vi "Build Metric Values.vi"(7 "TimingEngine":T1, 8 "error in (no error)":errorcluster, 10 "Waveform Array":sgl[][](array[numeric]), 11 "DAQ Task":refnum<class "DAQ Task.lvclass">) -> (0 "error out":errorcluster, 1 "Modbus Values":dbl[](array[numeric]), 2 "Ch Metrics":dbl[](array[numeric]), 3 "DAQ Task":refnum<class "DAQ Task.lvclass">)   [LabVIEW 2012, in "Data Acquisition.lvlib" / "DAQ Task.lvclass"]
uses:
  DAQ Task.lvclass
  Common/Controls/TE_Designator.ctl
  DAQ Task.lvclass/DAQ Task.ctl
  Measurements/Class Channel/Channel.lvclass
  Measurements/Class Channel/Read ToModBus.vi
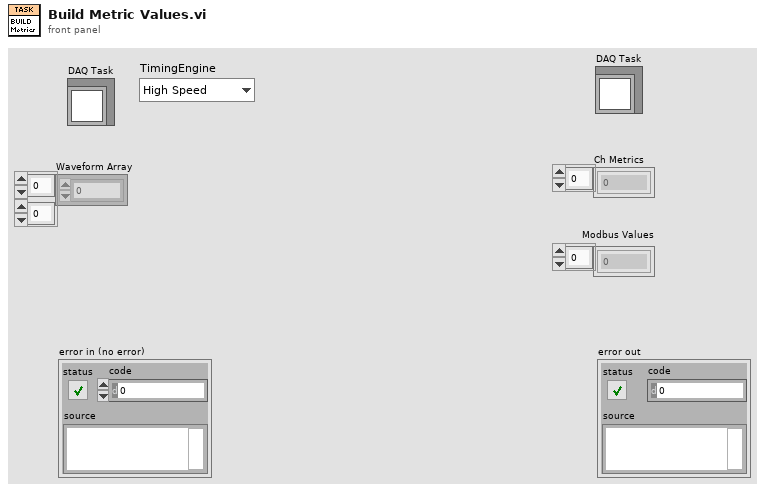
[diagram p1: front panel]
types:
  T1 = typedef "TE_Designator.ctl" = enum16{"High Speed", "Low Speed"}
  T2 = typedef "Group Timing Info.ctl" = cluster{"Rate":dbl, "ReadBlk":i32}
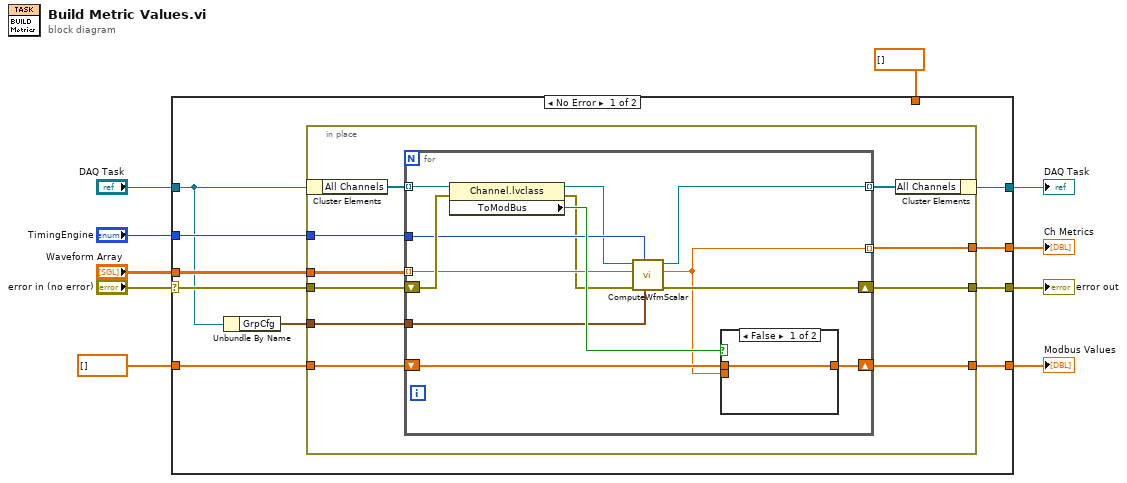
[diagram p0: block diagram]
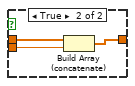
[diagram p2: hidden frame]
diagram:
  n1 = case shown="No Error" "error in (no error)" {
    selector: "error in (no error)" -> [w18 w50]
    tunnel: [w16 w48] -> w10
    tunnel: "Waveform Array" -> [w20 _]
    tunnel: "DAQ Task" -> [w12 w49]
    tunnel: [w15 w49] -> w7
    tunnel: [w19 w50] -> w6
    tunnel: "TimingEngine" -> [w17 _]
    tunnel: dbl[] [] -> [_ w48]
    tunnel: dbl[] [] -> [w14 _]
    tunnel: [w13 w48] -> w1
    frame No Error {
      n2 = Unbundle By Name(w12) -> ("GrpCfg"=w11:T2)
      n3 = in-place {
        in-place-border: w20 -> [w30]
        in-place-border: [w29] -> w19
        in-place-border: w18 -> [w28]
        in-place-border: w17 -> [w27]
        in-place-border: [w26] -> w16
        in-place-border: w14 -> [w23]
        in-place-border: [w22] -> w13
        in-place-border: w11 -> [w21]
        n4 = in-place-cluster #1(w12) -> ("All Channels"=w25:refnum<class "Channel.lvclass">[])
        n5 = for {
          tunnel: w30 -> [w40] mode=indexing
          tunnel: w25 -> [w43] mode=indexing
          shift-right: [w33] -> w29
          shift-left: w28 -> [w42]
          tunnel: w27 -> [w39]
          tunnel: [w36] -> w24 mode=indexing
          tunnel: [w32] -> w26 mode=indexing
          shift-right: [w34] -> w22
          shift-left: w23 -> [w35]
          tunnel: w21 -> [w31]
          n6 = property class="Channel.lvclass"(reference=w43, error in=w42) -> (reference out=w37:refnum<class "Channel.lvclass">, error out=w38:errorcluster, "ToModBus"=w41:bool)
          n7 = call-dynamic "ComputeWfmScalar.vi"("GrpCfg"=w31, "Speed"=w39, "error in (no error)"=w38, "Y Array"=w40, "Channel in"=w37) -> ("error out"=w33:errorcluster, "Metric"=w32:dbl, "Channel Out"=w36:refnum<class "Channel.lvclass">)  [unwired: 4 in]
          n8 = case shown="False" w41 {
            tunnel: w35 -> [w44 w47]
            tunnel: [w44 w46] -> w34
            tunnel: w32 -> [_ w45]
            frame False {
            }
            frame True {
              n9 = Build Array (concatenate)(w47, w45) -> (w46:dbl[])
            }
          }
        }
        n10 = in-place-cluster #1("All Channels"=w24) -> (w15:refnum<class "DAQ Task.lvclass">)
      }
    }
    frame Error {
    }
  }
  "Ch Metrics" <- w10
  "error out" <- w6
  "DAQ Task" <- w7
  "Modbus Values" <- w1
